vi "DMSP_main_VI_BM.vi"(0 "Constants":T4={"step to ml"=1920.0, "BoardNum"=1, "PosA BitNum"=6, "PosB BitNum"=5, "Heat Pulse Delay (ms)"=0.0, "Heating Iterations"=8, "N rinses"=2, "Dissolution Time (s)"=120, "SpargeBit"=0, "Extra Milli-Q (ml)"=2.0, "Valco Port Number"=6, "BitNum (Thermocouple)"=0, "N syringe rinses"=2, "NaOH Vol (ml)"=2.0, "FanBit"=0}, 1 "Hydrolysis Countdown Refnum":refnum<vi>, 2 "Metadata":T1={"Local save location:"="C:\\Users\\bcamc\\OneDrive\\Desktop\\LabVIEW\\Test_metadata", "Cruise ID"="LaPerouse", "Sampling Timestamp"="2023-07-19 15:23:13", "Elution Timestamp"="2023-07-19 15:29:12", "GPS_Latitude"=-999.0, "GPS_Longitude"=-999.0, "DMS_std_conc"=0.0, "DMSP_std_conc"=0.0, "DMSO_std_conc"=0.0, "Std_index"=0.0, "Initial Trap Temp (oC)"=174.0, "Max Trap Temp (oC)"=174.0, "Final Trap Temp (oC)"=0.0, "Flow Rate (mL/min)"=0.0, "Comment"="", "GPS_Minute"=-999.0, "GPS_Day"=-999.0, "GPS_jd"=-999.0, "GPS_Hour"=-999.0, "GPS_Second"=-999.0, "GPS Baud"=4800.0, "COM Port (GPS)"="COM10", "Use GPS?"=FALSE, "Format Date"="%d-%d-%d"} {"GPS_Latitude" format="%_4g"; "GPS_Longitude" format="%_4g"; "GPS_jd" format="%_5g"; "Std_index" format="%.2g"; "DMSO_std_conc" format="%.2f"; "DMSP_std_conc" format="%.2f"; "DMS_std_conc" format="%.2f"}, 3 "Hydrolysis Progress Bar Refnum":refnum<vi>, 4 "Sparge Countdown Timer Refnum":refnum<vi>, 5 "Sample Params":T5={"DMS Sparge Time (min)"=7.0, "Elution Time (min)"=1.5, "COM port (16 Pos. Valve)"="COM10", "Trap Heating Time (ms)"=675.0, "COM Port (DC Power)"="COM11", "COM Port (Runze)"="COM12", "sample volume"=10.0, "DMSO Red. Duration (min)"=30.0, "Bypass sample handling (debugging)"=FALSE, "Reverse Reduction?"=FALSE, "Voltage (V)"="4.0", "DMSP Hydrolysis Time (min)"=13.0, "Total Vol. (mL)"=12.0, "Split DMSP sample?"=FALSE, "Remove DMSP vol. (mL)"=4.0, "Extra Burn-off"=FALSE}, 6 "Sparging Progress Bar Refnum":refnum<vi>, 7 "Pump Parameters":T3={"Speed 1"="100", "Speed 2"="250", "Speed 3"="450", "Speed 4"="250", "UW/Sample"="5", "Sparge"="2", "Std"="4", "Waste"="15", "Air"="14", "Milli-Q"="1", "H2SO4"="6", "NaOH"="3", "Catalyst"="7", "Cell (H+ side)"="8", "Cell (sample side)"="9", "NaCl"="11"}, 9 "Mode Selection":T2(ring), 10 "Elution Countdown Timer Refnum":refnum<vi>, 11 "Analysis Type":T6(ring)=enum."DMS/P", 12 "Current Analyte Refnum":refnum<vi>, 14 "Temp Refnum":refnum<vi>, 15 "Elution Progress Bar Refnum":refnum<vi>) -> ()   [LabVIEW 2021]
uses:
  SubVIs/Timestamps_global.vi
  SubVIs/Refnum_control_global_BM.vi
  SubVIs/DMSP-related/Hydrolysis_stop.vi
  SubVIs/DMS-related/Sparge_stop.vi
  SubVIs/Plot_trap_heating_global_BM.vi
  SubVIs/DMS-related/Elution_stop.vi
  SubVIs/DMSO-related/Temp_global_BM.vi
panel:
  out "Current Analyte":string
  out "Hydrolysis Countdown (min)":dbl format="%.2g"
  out "Hydrolysis Progress Bar":u8(slide)=100 scale=0.0..100.0
  out "Drying Flow":bool
  out "Heating":bool
  in  "Error in":errorcluster
  out "Sparge Countdown (min)":dbl format="%.2g"
  out "Sparging Progress Bar":u8(slide)=100 scale=0.0..100.0
  out "Temp (oC)":i32=174
  out "Error out":errorcluster
  out "Elution Countdown (min)":dbl format="%.2f"
  out "Sparging":bool
  out "Elution Progress Bar":u8(slide)=100 scale=0.0..100.0
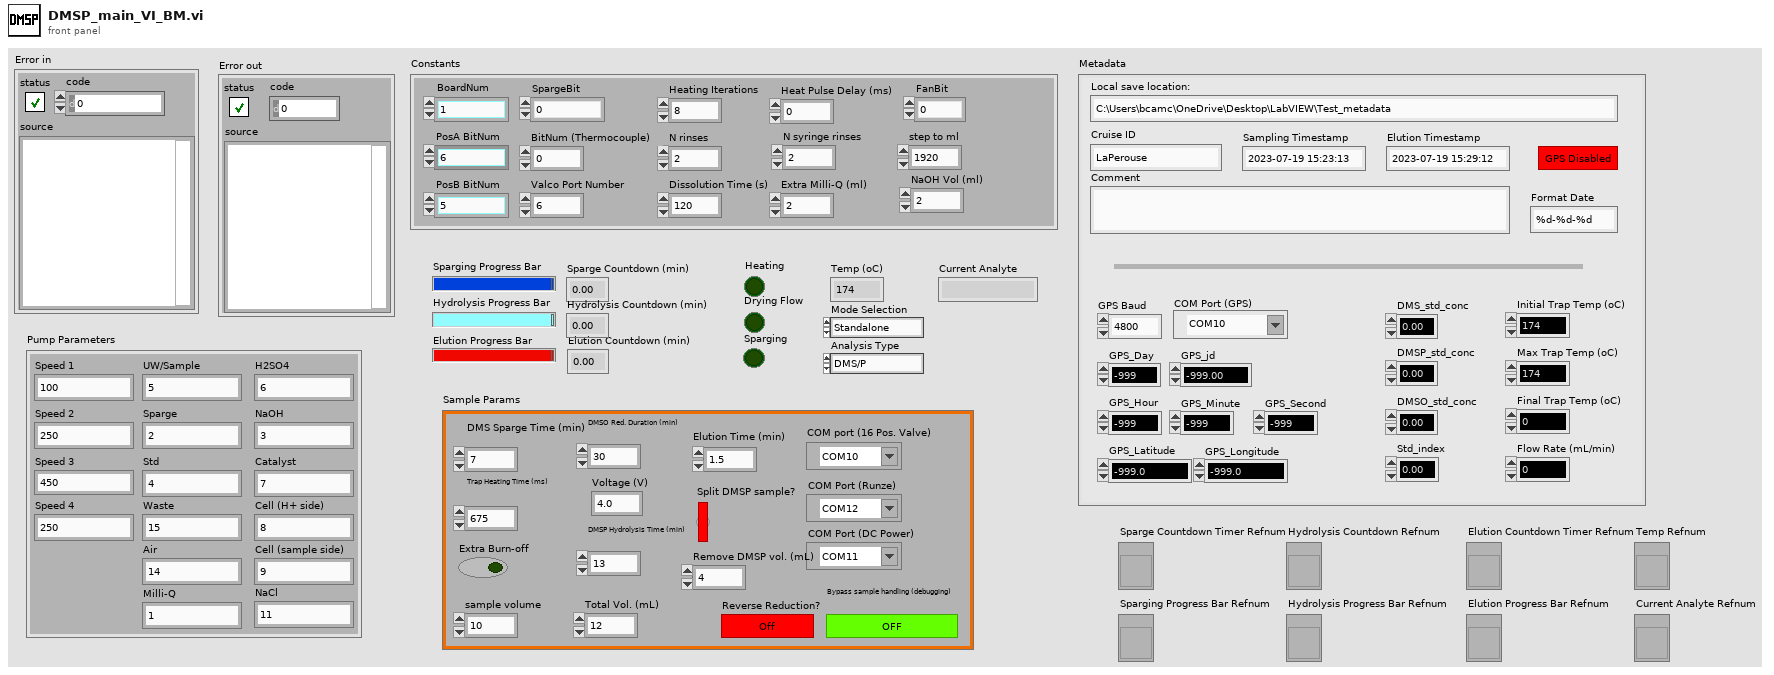
[diagram p1: front panel]
types:
  T1 = cluster{"Local save location:":string, "Cruise ID":string, "Sampling Timestamp":string, "Elution Timestamp":string, "GPS_Latitude":dbl, "GPS_Longitude":dbl, "DMS_std_conc":dbl, "DMSP_std_conc":dbl, "DMSO_std_conc":dbl, "Std_index":dbl, "Initial Trap Temp (oC)":dbl, "Max Trap Temp (oC)":dbl, "Final Trap Temp (oC)":dbl, "Flow Rate (mL/min)":dbl, "Comment":string, "GPS_Minute":dbl, "GPS_Day":dbl, "GPS_jd":dbl, "GPS_Hour":dbl, "GPS_Second":dbl, "GPS Baud":dbl, "COM Port (GPS)":refnum<visa-resource-name>, "Use GPS?":bool, "Format Date":string}
  T2 = enum16{"Standalone", "Analysis", "Standard Curve", "Point Std"}
  T3 = cluster{"Speed 1":string, "Speed 2":string, "Speed 3":string, "Speed 4":string, "UW/Sample":string, "Sparge":string, "Std":string, "Waste":string, "Air":string, "Milli-Q":string, "H2SO4":string, "NaOH":string, "Catalyst":string, "Cell (H+ side)":string, "Cell (sample side)":string, "NaCl":string}
  T4 = cluster{"step to ml":dbl, "BoardNum":u32, "PosA BitNum":u32, "PosB BitNum":u32, "Heat Pulse Delay (ms)":dbl, "Heating Iterations":i32, "N rinses":i32, "Dissolution Time (s)":u32, "SpargeBit":u32, "Extra Milli-Q (ml)":dbl, "Valco Port Number":i32, "BitNum (Thermocouple)":u32, "N syringe rinses":i32, "NaOH Vol (ml)":dbl, "FanBit":u32}
  T5 = cluster{"DMS Sparge Time (min)":dbl, "Elution Time (min)":dbl, "COM port (16 Pos. Valve)":refnum<visa-resource-name>, "Trap Heating Time (ms)":dbl, "COM Port (DC Power)":refnum<visa-resource-name>, "COM Port (Runze)":refnum<visa-resource-name>, "sample volume":dbl, "DMSO Red. Duration (min)":dbl, "Bypass sample handling (debugging)":bool, "Reverse Reduction?":bool, "Voltage (V)":string, "DMSP Hydrolysis Time (min)":dbl, "Total Vol. (mL)":dbl, "Split DMSP sample?":bool, "Remove DMSP vol. (mL)":dbl, "Extra Burn-off":bool}
  T6 = enum16{"DMS Only", "DMS/O", "DMS/P", "DMS/O/P", "DMSO Only"}
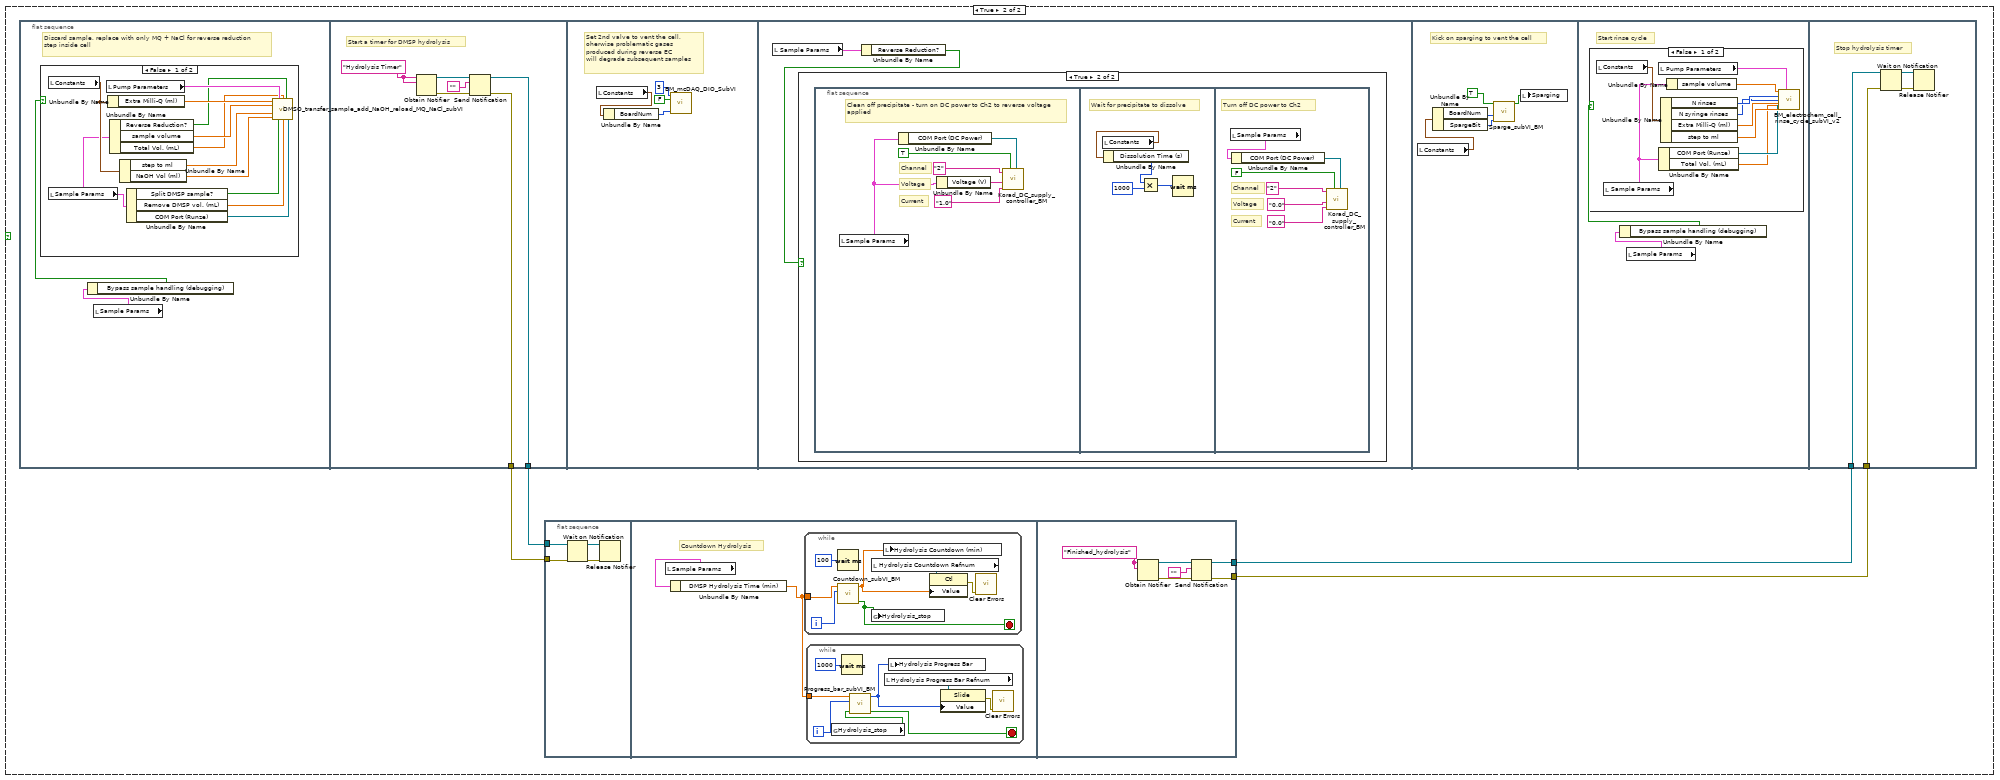
[diagram p10: hidden frame]
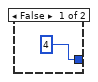
[diagram p15: hidden frame]
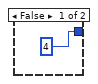
[diagram p17: hidden frame]
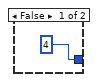
[diagram p20: hidden frame]
diagram:
  n1 = flat-sequence {
    tunnel: [w327] -> w6
    tunnel: [w326] -> w5
    tunnel: [w321] -> w2
    tunnel: [w320] -> w1
    tunnel: [w343] -> w10
    tunnel: [w348] -> w9
    tunnel: w10 -> [w348]
    tunnel: w9 -> [w352]
    tunnel: [w377] -> w8
    tunnel: w8 -> [w387]
    tunnel: [w387] -> w4
    tunnel: w4 -> [w409]
    tunnel: [w409] -> w3
    tunnel: w3 -> [w416]
    tunnel: [w416] -> w7
    tunnel: w7 -> [w424]
    frame #0 {
      w20 = "DMSP" ("Current Analysis")
      # "Update sampling / elution times from DMS VI"
      # "If run on OSSCAR, set the flow path back to the sparge chamber"
      # "Indicate for user to track"
      # "Initalize syringe pump"
      n2 = local read "Constants"() -> (w18:T4)
      n3 = global read "Timestamps_global.vi" "Sampling Timestamp"() -> (w11:string)
      n4 = global read "Timestamps_global.vi" "Elution Timestamp"() -> (w12:string)
      n5 = Unbundle By Name(w18) -> ("BoardNum"=w16:u32)
      n6 = local read "Sample Params"() -> (w22:T5)
      n7 = Unbundle By Name(w22) -> ("Bypass sample handling (debugging)"=w23:bool)
      n8 = case shown="False" w23 {
        frame False {
          n9 = local read "Sample Params"() -> (w26:T5)
          n10 = Unbundle By Name(w26) -> ("COM Port (Runze)"=w27:refnum<visa-resource-name>)
          n11 = call "BM_Runze_Syringe_Pump_Controller.vi"("Initialize Plunger?"=TRUE ("Initialize?"), "COM Port (Runze)"=w27, "Enter Command"="") -> ()  [unwired: 6 in, 3 out]
        }
        frame True {
        }
      }
      n12 = local read "Current Analyte Refnum"() -> (w21:refnum<vi>)
      n13 = local write "Current Analyte"(w20) -> ()
      n14 = Equal?(x=u32 0, y=w16) -> (x = y?=w17:bool)
      n15 = property class="Ctl"(reference=w21, "Value"=w20) -> (error out=w19:errorcluster)  [unwired: 1 in, 1 out]
      n16 = case shown="True" w17 {
        tunnel: w16 -> [_ w24]
        frame False {
        }
        frame True {
          n17 = call "EC_switch_flow_path_subVI_BM.vi"("BoardNum"=w24, "Switch Flow Path"=FALSE) -> ()  [unwired: 10 in]
        }
      }
      n18 = local read "Metadata"() -> (w14:T1)
      n19 = Bundle By Name(cluster=w14, "Sampling Timestamp"=w11, "Elution Timestamp"=w12) -> (w13:T1)
      n20 = call <vilib>:"Clear Errors.vi"("error in (no error)"=w19) -> ()  [unwired: 5 in, 2 out]
      n21 = local write "Metadata"(w13) -> ()
    }
    frame #1 {
      # "Turn on sparging."
      # "Switch Valco valve to position A: load."
      # "Begin sample handling"
      n22 = local read "Constants"() -> (w37:T4)
      n23 = Unbundle By Name(w37) -> ("PosA BitNum"=w36:u32, "PosB BitNum"=w35:u32, "BoardNum"=w34:u32, "SpargeBit"=w33:u32)
      n24 = Equal?(x=w34, y=u32 1) -> (x = y?=w39:bool)
      n25 = case shown="True" w39 {
        tunnel: w34 -> [_ w44]
        frame False {
        }
        frame True {
          # "Switch to sample port"
          # "Start Drying Flow"
          n26 = local read "Constants"() -> (w42:T4)
          n27 = local read "Sample Params"() -> (w40:T5)
          n28 = Unbundle By Name(w40) -> ("COM port (16 Pos. Valve)"=w41:refnum<visa-resource-name>)
          n29 = Unbundle By Name(w42) -> ("Valco Port Number"=w43:i32)
          n30 = call "BM_mcDAQ_DIO_SubVI.vi"("BoardNum"=w44, "BitValue"=TRUE, "BitNum"=4) -> ("Control out"=w47:bool)  [unwired: 8 in]
          n31 = local write "Drying Flow"(w47) -> ()
          n32 = call "16portvalco_subVI_BM.vi"("COM Port (16 Pos. Valve)"=w41, "Port Number"=w43) -> ()  [unwired: 9 in, 1 out]
        }
      }
      n33 = call "Sparge_subVI_BM.vi"("BitNum"=w33, "BoardNum"=w34, "Sparge now"=TRUE) -> ("Sparging"=w38:bool)  [unwired: 8 in]
      n34 = local write "Sparging"(w38) -> ()
      n35 = call "Switch_Valco_6port_subVI_BM.vi"("Load (T) or Inject (F)"=TRUE, "PosA BitNum"=w36, "PosB BitNum"=w35, "BoardNum"=w34) -> ()  [unwired: 6 in, 1 out]
    }
    frame #2 {
      # "2 options here for sampling handling, based on the analysis type:\n1. \"DMS/O/P\" mode - transfer sample to sparger, add NaOH to sparger, start a timer, then either clean off precipitate + rinse cell or just rinse cell, while waiting for hydrolysis to finish\n2. \"DMS/P\" mode - Run DMS VI, split sample (optional), then add NaOH\nOther modes are N/A"
      n36 = local read "Analysis Type"() -> (w50:T6)
      n37 = Equal?(x=w50, y=T6."DMS/O/P") -> (x = y?=w49:bool)
      n38 = case shown="False" w49 {
        frame False {
          n39 = local read "Analysis Type"() -> (w52:T6)
          n40 = Equal?(x=w52, y=T6."DMS/P") -> (x = y?=w51:bool)
          n41 = case shown="True" w51 {
            frame False {
              # "Analysis mode is set to either \"DMS Only\", \"DMSO Only\" or \"DMS/O\", all of which are N/A here"
            }
            frame True {
              n42 = flat-sequence {
                tunnel: [w180] -> w55
                tunnel: [w179] -> w54
                tunnel: w57 -> [w194]
                tunnel: w56 -> [w193]
                frame #0 {
                  # "Sample handle / sparge off DMS first"
                  n43 = while {
                    stop <- w105 stop-if-true
                    # "Update refnums from DMS subVI - this ensures they pass through to main OSSCAR VI"
                    n44 = local read "Elution Countdown Timer Refnum"() -> (w100:refnum<vi>)
                    n45 = local read "Sparge Countdown Timer Refnum"() -> (w112:refnum<vi>)
                    n46 = local read "Elution Countdown Timer Refnum"() -> (w103:refnum<vi>)
                    n47 = local read "Sparging Progress Bar Refnum"() -> (w115:refnum<vi>)
                    n48 = local read "Elution Countdown (min)"() -> (w101:dbl)
                    n49 = local read "Sparge Countdown (min)"() -> (w113:dbl)
                    n50 = local read "Sparging Progress Bar"() -> (w114:u8)
                    n51 = local read "Elution Progress Bar"() -> (w102:u8)
                    n52 = local read "Temp Refnum"() -> (w109:refnum<vi>)
                    n53 = global read "Refnum_control_global_BM.vi" "Refnum_control"() -> (w107:bool)
                    n54 = local read "Temp (oC)"() -> (w108:i32)
                    n55 = property class="Slide"(reference=w115, "Value"=w114) -> (error out=w116:errorcluster)  [unwired: 1 in, 1 out]
                    n56 = property class="Ctl"(reference=w100, "Value"=w101) -> (error out=w99:errorcluster)  [unwired: 1 in, 1 out]
                    n57 = property class="Ctl"(reference=w109, "Value"=w108) -> (error out=w110:errorcluster)  [unwired: 1 in, 1 out]
                    n58 = property class="Ctl"(reference=w112, "Value"=w113) -> (error out=w111:errorcluster)  [unwired: 1 in, 1 out]
                    n59 = property class="Ctl"(reference=w103, "Value"=w102) -> (error out=w104:errorcluster)  [unwired: 1 in, 1 out]
                    n60 = Equal?(x=w107, y=TRUE) -> (x = y?=w105:bool)
                    n61 = call <vilib>:"Clear Errors.vi"("error in (no error)"=w116) -> ()  [unwired: 5 in, 2 out]
                    n62 = call <vilib>:"Clear Errors.vi"("error in (no error)"=w99) -> ()  [unwired: 5 in, 2 out]
                    n63 = call <vilib>:"Clear Errors.vi"("error in (no error)"=w110) -> ()  [unwired: 5 in, 2 out]
                    n64 = Wait (ms)(milliseconds to wait=u32 100) -> ()  [unwired: 1 out]
                    n65 = call <vilib>:"Clear Errors.vi"("error in (no error)"=w111) -> ()  [unwired: 5 in, 2 out]
                    n66 = call <vilib>:"Clear Errors.vi"("error in (no error)"=w104) -> ()  [unwired: 5 in, 2 out]
                  }
                  n67 = local read "Pump Parameters"() -> (w95:T3)
                  n68 = local read "Mode Selection"() -> (w87:T2)
                  n69 = local read "Sample Params"() -> (w96:T5)
                  n70 = local read "Analysis Type"() -> (w94:T6)
                  n71 = local read "Constants"() -> (w97:T4)
                  n72 = local read "Metadata"() -> (w93:T1)
                  n73 = control-ref of="Elution Countdown (min)"() -> (w90:refnum<vi>)
                  n74 = control-ref of="Temp (oC)"() -> (w89:refnum<vi>)
                  n75 = control-ref of="Current Analyte"() -> (w85:refnum<vi>)
                  n76 = control-ref of="Elution Progress Bar"() -> (w91:refnum<vi>)
                  n77 = control-ref of="Sparge Countdown (min)"() -> (w92:refnum<vi>)
                  n78 = control-ref of="Sparging Progress Bar"() -> (w88:refnum<vi>)
                  n79 = call "DMS_main_VI_BM.vi"("Constants"=w97, "Metadata"=w93, "Skip sample handling"=FALSE, "Sparging Countdown Timer Refnum"=w92, "Sample Params"=w96, "Sparging Progress Bar Refnum"=w88, "Pump Parameters"=w95, "Mode Selection"=w87, "Elution Countdown Timer Refnum"=w90, "Analysis Type"=w94, "Current Analyte Refnum"=w85, "Temp Refnum"=w89, "Elution Progress Bar Refnum"=w91) -> ()  [unwired: 3 in]
                }
                frame #1 {
                  # "Optional: If splitting DMSP sample to reduce ion counts on the detector, remove chosen vol. here and send to waste"
                  n80 = local read "Sample Params"() -> (w118:T5)
                  n81 = Unbundle By Name(w118) -> ("Split DMSP sample?"=w117:bool)
                  n82 = case shown="True" w117 {
                    frame False {
                      # "If not splitting sample, continue with analysis"
                    }
                    frame True {
                      n83 = local read "Sample Params"() -> (w124:T5)
                      n84 = local read "Pump Parameters"() -> (w136:T3)
                      n85 = local read "Constants"() -> (w122:T4)
                      n86 = Unbundle By Name(w124) -> ("Remove DMSP vol. (mL)"=w125:dbl)
                      n87 = Unbundle By Name(w124) -> ("Remove DMSP vol. (mL)"=w126:dbl)
                      n88 = Unbundle By Name(w122) -> ("step to ml"=w121:dbl)
                      n89 = Unbundle By Name(w122) -> ("step to ml"=w123:dbl)
                      n90 = Multiply(x=w125, y=w121) -> (x*y=w146:dbl)
                      n91 = Multiply(x=w126, y=w123) -> (x*y=w148:dbl)
                      n92 = Unbundle By Name(w136) -> ("Speed 2"=w139:string)
                      n93 = Unbundle By Name(w136) -> ("Speed 1"=w149:string)
                      n94 = Unbundle By Name(w136) -> ("Sparge"=w135:string)
                      n95 = Unbundle By Name(w136) -> ("Waste"=w134:string)
                      n96 = Number To Decimal String(number=w148) -> (decimal integer string=w147:string)  [unwired: 1 out]
                      n97 = Number To Decimal String(number=w146) -> (decimal integer string=w145:string)  [unwired: 1 out]
                      n98 = Concatenate Strings("V", w149) -> (w144:string)
                      n99 = Concatenate Strings("O", w135) -> (w143:string)
                      n100 = Concatenate Strings("P", w147) -> (w142:string)
                      n101 = Concatenate Strings("O", w134) -> (w141:string)
                      n102 = Concatenate Strings("D", w145) -> (w137:string)
                      n103 = Concatenate Strings("V", w139) -> (w138:string)
                      n104 = local read "Sample Params"() -> (w119:T5)
                      n105 = Unbundle By Name(w119) -> ("COM Port (Runze)"=w120:refnum<visa-resource-name>)
                      n106 = Concatenate Strings(w144, w143, w142, w141, w138, w137) -> (w140:string)
                      n107 = call "BM_Runze_Syringe_Pump_Controller.vi"("Initialize Plunger?"=FALSE ("Initialize?"), "COM Port (Runze)"=w120, "Enter Command"=w140) -> ()  [unwired: 6 in, 3 out]
                    }
                  }
                }
                frame #2 {
                  # "Turn on sparging."
                  # "Switch Valco valve to position A: load."
                  # "Begin sample handling"
                  n108 = local read "Constants"() -> (w158:T4)
                  n109 = Unbundle By Name(w158) -> ("PosA BitNum"=w157:u32, "PosB BitNum"=w156:u32, "BoardNum"=w155:u32, "SpargeBit"=w154:u32)
                  n110 = Equal?(x=w155, y=u32 1) -> (x = y?=w150:bool)
                  n111 = case shown="True" w150 {
                    tunnel: w155 -> [_ w164]
                    frame False {
                    }
                    frame True {
                      # "Switch to sample port"
                      # "Start Drying Flow"
                      n112 = local read "Constants"() -> (w162:T4)
                      n113 = local read "Sample Params"() -> (w160:T5)
                      n114 = Unbundle By Name(w160) -> ("COM port (16 Pos. Valve)"=w161:refnum<visa-resource-name>)
                      n115 = Unbundle By Name(w162) -> ("Valco Port Number"=w163:i32)
                      n116 = call "BM_mcDAQ_DIO_SubVI.vi"("BoardNum"=w164, "BitValue"=TRUE, "BitNum"=4) -> ("Control out"=w167:bool)  [unwired: 8 in]
                      n117 = local write "Drying Flow"(w167) -> ()
                      n118 = call "16portvalco_subVI_BM.vi"("COM Port (16 Pos. Valve)"=w161, "Port Number"=w163) -> ()  [unwired: 9 in, 1 out]
                    }
                  }
                  n119 = call "Sparge_subVI_BM.vi"("BitNum"=w154, "BoardNum"=w155, "Sparge now"=TRUE) -> ("Sparging"=w159:bool)  [unwired: 8 in]
                  n120 = local write "Sparging"(w159) -> ()
                  n121 = call "Switch_Valco_6port_subVI_BM.vi"("Load (T) or Inject (F)"=TRUE, "PosA BitNum"=w157, "PosB BitNum"=w156, "BoardNum"=w155) -> ()  [unwired: 6 in, 1 out]
                }
                frame #3 {
                  # "Add NaOH to sparger"
                  n122 = local read "Sample Params"() -> (w168:T5)
                  n123 = Unbundle By Name(w168) -> ("Bypass sample handling (debugging)"=w169:bool)
                  n124 = case shown="False" w169 {
                    frame False {
                      n125 = local read "Sample Params"() -> (w173:T5)
                      n126 = local read "Sample Params"() -> (w175:T5)
                      n127 = local read "Constants"() -> (w177:T4)
                      n128 = local read "Pump Parameters"() -> (w178:T3)
                      n129 = Unbundle By Name(w177) -> ("step to ml"=w176:dbl, "NaOH Vol (ml)"=w171:dbl)
                      n130 = Unbundle By Name(w173) -> ("COM Port (Runze)"=w172:refnum<visa-resource-name>)
                      n131 = Unbundle By Name(w175) -> ("sample volume"=w174:dbl, "Total Vol. (mL)"=w170:dbl)
                      n132 = call "DMSP_add_NaOH_BM.vi"("COM Port"=w172, "Pump Parameters"=w178, "NaOH Vol (mL)"=w171, "step to ml"=w176, "Total Vol. (mL)"=w170, "Sample Vol. (mL)"=w174) -> ()  [unwired: 6 in]
                    }
                    frame True {
                    }
                  }
                }
                frame #4 {
                  w181 = "Hydrolysis Timer"
                  # "Start a timer for DMSP hydrolysis"
                  n133 = Obtain Notifier(name (unnamed)=w181, notification data type=w181) -> (notifier out=w183:refnum<notifier>, error out=w184:errorcluster)  [unwired: 2 in, 1 out]
                  n134 = Send Notification(notification="", notifier=w183, error in (no error)=w184) -> (notifier out=w180:refnum<notifier>, error out=w179:errorcluster)
                }
                frame #5 {
                  # "Rinse Syringe"
                  n135 = local read "Sample Params"() -> (w185:T5)
                  n136 = Unbundle By Name(w185) -> ("Bypass sample handling (debugging)"=w186:bool)
                  n137 = case shown="False" w186 {
                    frame False {
                      n138 = local read "Sample Params"() -> (w189:T5)
                      n139 = local read "Constants"() -> (w191:T4)
                      n140 = local read "Pump Parameters"() -> (w192:T3)
                      n141 = Unbundle By Name(w191) -> ("step to ml"=w190:dbl, "N syringe rinses"=w187:i32)
                      n142 = Unbundle By Name(w189) -> ("COM Port (Runze)"=w188:refnum<visa-resource-name>)
                      n143 = call "Rinse_syringe_subVI_BM.vi"("COM Port"=w188, "Pump Parameters"=w192, "N syringe rinses"=w187, "step to ml"=w190) -> ()  [unwired: 8 in]
                    }
                    frame True {
                    }
                  }
                }
                frame #6 {
                  # "Stop hydrolysis timer"
                  n144 = Wait on Notification(notifier=w194, error in (no error)=w193) -> (notifier out=w195:refnum<notifier>, error out=w196:errorcluster)  [unwired: 4 out]
                  n145 = Release Notifier(notifier=w195, error in (no error)=w196) -> ()  [unwired: 1 in, 3 out]
                }
              }
              n146 = flat-sequence {
                tunnel: w54 -> [w58]
                tunnel: w55 -> [w59]
                tunnel: [w80] -> w57
                tunnel: [w79] -> w56
                frame #0 {
                  n147 = Wait on Notification(notifier=w59, error in (no error)=w58) -> (notifier out=w61:refnum<notifier>, error out=w60:errorcluster)  [unwired: 4 out]
                  n148 = Release Notifier(notifier=w61, error in (no error)=w60) -> ()  [unwired: 1 in, 3 out]
                }
                frame #1 {
                  # "Countdown Hydrolysis"
                  n149 = local read "Sample Params"() -> (w63:T5)
                  n150 = Unbundle By Name(w63) -> ("DMSP Hydrolysis Time (min)"=w62:dbl)
                  n151 = while {
                    tunnel: w62 -> [w77]
                    i -> [w76]
                    stop <- w75 stop-if-true
                    n152 = Wait (ms)(milliseconds to wait=u32 100) -> ()  [unwired: 1 out]
                    n153 = call "Countdown_subVI_BM.vi"("Current Iteration"=w76, "Runtime (min)"=w77) -> ("Global Stop"=w75:bool, "Countdown Timer (min)"=w74:dbl)  [unwired: 8 in]
                    n154 = global write "Hydrolysis_stop.vi" "Hydrolysis_stop"(w75) -> ()
                    n155 = local read "Hydrolysis Countdown Refnum"() -> (w72:refnum<vi>)
                    n156 = local write "Hydrolysis Countdown (min)"(w74) -> ()
                    n157 = property class="Ctl"(reference=w72, "Value"=w74) -> (error out=w73:errorcluster)  [unwired: 1 in, 1 out]
                    n158 = call <vilib>:"Clear Errors.vi"("error in (no error)"=w73) -> ()  [unwired: 5 in, 2 out]
                  }
                  n159 = while {
                    tunnel: w62 -> [w70]
                    i -> [w69]
                    stop <- w67 stop-if-true
                    n160 = global read "Hydrolysis_stop.vi" "Hydrolysis_stop"() -> (w68:bool)
                    n161 = Wait (ms)(milliseconds to wait=u32 1000) -> ()  [unwired: 1 out]
                    n162 = call "Progress_bar_subVI_BM.vi"("Global Stop"=w68, "Current Iteration"=w69, "Runtime (min)"=w70) -> ("Loop Stop"=w67:bool, "Progress Bar"=w66:u8)  [unwired: 7 in]
                    n163 = local read "Hydrolysis Progress Bar Refnum"() -> (w64:refnum<vi>)
                    n164 = local write "Hydrolysis Progress Bar"(w66) -> ()
                    n165 = property class="Slide"(reference=w64, "Value"=w66) -> (error out=w65:errorcluster)  [unwired: 1 in, 1 out]
                    n166 = call <vilib>:"Clear Errors.vi"("error in (no error)"=w65) -> ()  [unwired: 5 in, 2 out]
                  }
                }
                frame #2 {
                  w83 = "Finished_hydrolysis"
                  n167 = Obtain Notifier(name (unnamed)=w83, notification data type=w83) -> (notifier out=w81:refnum<notifier>, error out=w82:errorcluster)  [unwired: 2 in, 1 out]
                  n168 = Send Notification(notification="", notifier=w81, error in (no error)=w82) -> (notifier out=w80:refnum<notifier>, error out=w79:errorcluster)
                }
              }
            }
          }
        }
        frame True {
          n169 = flat-sequence {
            tunnel: [w244] -> w200
            tunnel: [w243] -> w199
            tunnel: w197 -> [w288]
            tunnel: w198 -> [w287]
            frame #0 {
              # "Discard sample, replace with only MQ + NaCl for reverse reduction step inside cell"
              n170 = local read "Sample Params"() -> (w229:T5)
              n171 = Unbundle By Name(w229) -> ("Bypass sample handling (debugging)"=w228:bool)
              n172 = case shown="False" w228 {
                frame False {
                  n173 = local read "Constants"() -> (w239:T4)
                  n174 = local read "Sample Params"() -> (w237:T5)
                  n175 = local read "Pump Parameters"() -> (w241:T3)
                  n176 = Unbundle By Name(w239) -> ("Extra Milli-Q (ml)"=w240:dbl)
                  n177 = Unbundle By Name(w237) -> ("Reverse Reduction?"=w233:bool, "sample volume"=w238:dbl, "Total Vol. (mL)"=w232:dbl)
                  n178 = Unbundle By Name(w239) -> ("step to ml"=w235:dbl, "NaOH Vol (ml)"=w234:dbl)
                  n179 = Unbundle By Name(w237) -> ("Split DMSP sample?"=w230:bool, "Remove DMSP vol. (mL)"=w231:dbl, "COM Port (Runze)"=w236:refnum<visa-resource-name>)
                  n180 = call "DMSO_transfer_sample_add_NaOH_reload_MQ_NaCl_subVI.vi"("Extra Milli-Q (ml)"=w240, "Pump Parameters"=w241, "Total Vol. (mL)"=w232, "Reverse Reduction?"=w233, "Sample Vol. (mL)"=w238, "step to ml"=w235, "NaOH Vol (mL)"=w234, "Split DMSP sample?"=w230, "Remove DMSP vol. (mL)"=w231, "COM Port"=w236) -> ()  [unwired: 6 in]
                }
                frame True {
                }
              }
            }
            frame #1 {
              w245 = "Hydrolysis Timer"
              # "Start a timer for DMSP hydrolysis"
              n181 = Obtain Notifier(name (unnamed)=w245, notification data type=w245) -> (notifier out=w246:refnum<notifier>, error out=w247:errorcluster)  [unwired: 2 in, 1 out]
              n182 = Send Notification(notification="", notifier=w246, error in (no error)=w247) -> (notifier out=w243:refnum<notifier>, error out=w244:errorcluster)
            }
            frame #2 {
              # "Set 2nd valve to vent the cell,\noherwise problematic gases\nproduced during reverse EC \nwill degrade subsequent samples"
              n183 = local read "Constants"() -> (w248:T4)
              n184 = Unbundle By Name(w248) -> ("BoardNum"=w251:u32)
              n185 = call "BM_mcDAQ_DIO_SubVI.vi"("BoardNum"=w251, "BitValue"=FALSE, "BitNum"=u32 3) -> ()  [unwired: 8 in, 1 out]
            }
            frame #3 {
              n186 = local read "Sample Params"() -> (w253:T5)
              n187 = Unbundle By Name(w253) -> ("Reverse Reduction?"=w252:bool)
              n188 = case shown="True" w252 {
                frame False {
                  # "Skip to rinsing out the cell"
                }
                frame True {
                  n189 = flat-sequence {
                    frame #0 {
                      # "Channel"
                      # "Current"
                      # "Voltage"
                      # "Clean off precipitate - turn on DC power to Ch2 to reverse voltage applied"
                      n190 = local read "Sample Params"() -> (w254:T5)
                      n191 = Unbundle By Name(w254) -> ("COM Port (DC Power)"=w256:refnum<visa-resource-name>)
                      n192 = Unbundle By Name(w254) -> ("Voltage (V)"=w255:string)
                      n193 = call "Korad_DC_supply_controller_BM.vi"("COM Port"=w256, "Master Output Control"=TRUE ("Output Control"), "Current"="1.0" ("Ch2 Current"), "Voltage"=w255, "Channel"="2" ("Ch1 Voltage")) -> ()  [unwired: 7 in]
                    }
                    frame #1 {
                      # "Wait for precipitate to dissolve"
                      n194 = local read "Constants"() -> (w261:T4)
                      n195 = Unbundle By Name(w261) -> ("Dissolution Time (s)"=w260:u32)
                      n196 = Multiply(x=w260, y=u32 1000) -> (x*y=w263:u32)
                      n197 = Wait (ms)(milliseconds to wait=w263) -> ()  [unwired: 1 out]
                    }
                    frame #2 {
                      # "Channel"
                      # "Current"
                      # "Voltage"
                      # "Turn off DC power to Ch2"
                      n198 = local read "Sample Params"() -> (w265:T5)
                      n199 = Unbundle By Name(w265) -> ("COM Port (DC Power)"=w264:refnum<visa-resource-name>)
                      n200 = call "Korad_DC_supply_controller_BM.vi"("COM Port"=w264, "Master Output Control"=FALSE ("Output Control"), "Current"="0.0" ("Ch2 Current"), "Voltage"="0.0" ("Ch1 Voltage"), "Channel"="2" ("Ch1 Voltage")) -> ()  [unwired: 7 in]
                    }
                  }
                }
              }
            }
            frame #4 {
              # "Kick on sparging to vent the cell"
              n201 = local read "Constants"() -> (w272:T4)
              n202 = Unbundle By Name(w272) -> ("BoardNum"=w271:u32, "SpargeBit"=w270:u32)
              n203 = call "Sparge_subVI_BM.vi"("BitNum"=w270, "BoardNum"=w271, "Sparge now"=TRUE) -> ("Sparging"=w273:bool)  [unwired: 8 in]
              n204 = local write "Sparging"(w273) -> ()
            }
            frame #5 {
              # "Start rinse cycle"
              n205 = local read "Sample Params"() -> (w275:T5)
              n206 = Unbundle By Name(w275) -> ("Bypass sample handling (debugging)"=w276:bool)
              n207 = case shown="False" w276 {
                frame False {
                  n208 = local read "Constants"() -> (w283:T4)
                  n209 = local read "Sample Params"() -> (w280:T5)
                  n210 = local read "Pump Parameters"() -> (w286:T3)
                  n211 = Unbundle By Name(w280) -> ("COM Port (Runze)"=w281:refnum<visa-resource-name>, "Total Vol. (mL)"=w277:dbl)
                  n212 = Unbundle By Name(w283) -> ("N rinses"=w279:i32, "N syringe rinses"=w278:i32, "Extra Milli-Q (ml)"=w285:dbl, "step to ml"=w284:dbl)
                  n213 = Unbundle By Name(w280) -> ("sample volume"=w282:dbl)
                  n214 = call "BM_electrochem_cell_rinse_cycle_subVI_v2.vi"("Sample Volume"=w282, "Pump Parameters"=w286, "N cell rinses"=w279, "N syringe rinses"=w278, "Extra Milli-Q (ml)"=w285, "step to ml"=w284, "COM Port"=w281, "Total Vol. (mL)"=w277) -> ()  [unwired: 8 in]
                }
                frame True {
                }
              }
            }
            frame #6 {
              # "Stop hydrolysis timer"
              n215 = Wait on Notification(notifier=w287, error in (no error)=w288) -> (notifier out=w289:refnum<notifier>, error out=w290:errorcluster)  [unwired: 4 out]
              n216 = Release Notifier(notifier=w289, error in (no error)=w290) -> ()  [unwired: 1 in, 3 out]
            }
          }
          n217 = flat-sequence {
            tunnel: w200 -> [w201]
            tunnel: w199 -> [w202]
            tunnel: [w223] -> w198
            tunnel: [w222] -> w197
            frame #0 {
              n218 = Wait on Notification(notifier=w202, error in (no error)=w201) -> (notifier out=w204:refnum<notifier>, error out=w203:errorcluster)  [unwired: 4 out]
              n219 = Release Notifier(notifier=w204, error in (no error)=w203) -> ()  [unwired: 1 in, 3 out]
            }
            frame #1 {
              # "Countdown Hydrolysis"
              n220 = local read "Sample Params"() -> (w206:T5)
              n221 = Unbundle By Name(w206) -> ("DMSP Hydrolysis Time (min)"=w205:dbl)
              n222 = while {
                tunnel: w205 -> [w220]
                i -> [w219]
                stop <- w218 stop-if-true
                n223 = Wait (ms)(milliseconds to wait=u32 100) -> ()  [unwired: 1 out]
                n224 = call "Countdown_subVI_BM.vi"("Current Iteration"=w219, "Runtime (min)"=w220) -> ("Global Stop"=w218:bool, "Countdown Timer (min)"=w217:dbl)  [unwired: 8 in]
                n225 = global write "Hydrolysis_stop.vi" "Hydrolysis_stop"(w218) -> ()
                n226 = local read "Hydrolysis Countdown Refnum"() -> (w215:refnum<vi>)
                n227 = local write "Hydrolysis Countdown (min)"(w217) -> ()
                n228 = property class="Ctl"(reference=w215, "Value"=w217) -> (error out=w216:errorcluster)  [unwired: 1 in, 1 out]
                n229 = call <vilib>:"Clear Errors.vi"("error in (no error)"=w216) -> ()  [unwired: 5 in, 2 out]
              }
              n230 = while {
                tunnel: w205 -> [w213]
                i -> [w212]
                stop <- w210 stop-if-true
                n231 = global read "Hydrolysis_stop.vi" "Hydrolysis_stop"() -> (w211:bool)
                n232 = Wait (ms)(milliseconds to wait=u32 1000) -> ()  [unwired: 1 out]
                n233 = call "Progress_bar_subVI_BM.vi"("Global Stop"=w211, "Current Iteration"=w212, "Runtime (min)"=w213) -> ("Loop Stop"=w210:bool, "Progress Bar"=w209:u8)  [unwired: 7 in]
                n234 = local read "Hydrolysis Progress Bar Refnum"() -> (w207:refnum<vi>)
                n235 = local write "Hydrolysis Progress Bar"(w209) -> ()
                n236 = property class="Slide"(reference=w207, "Value"=w209) -> (error out=w208:errorcluster)  [unwired: 1 in, 1 out]
                n237 = call <vilib>:"Clear Errors.vi"("error in (no error)"=w208) -> ()  [unwired: 5 in, 2 out]
              }
            }
            frame #2 {
              w226 = "Finished_hydrolysis"
              n238 = Obtain Notifier(name (unnamed)=w226, notification data type=w226) -> (notifier out=w224:refnum<notifier>, error out=w225:errorcluster)  [unwired: 2 in, 1 out]
              n239 = Send Notification(notification="", notifier=w224, error in (no error)=w225) -> (notifier out=w223:refnum<notifier>, error out=w222:errorcluster)
            }
          }
        }
      }
    }
    frame #3 {
      # "Countdown sparging"
      n240 = local read "Sample Params"() -> (w291:T5)
      n241 = Unbundle By Name(w291) -> ("DMS Sparge Time (min)"=w292:dbl)
      n242 = while {
        tunnel: w292 -> [w306]
        i -> [w305]
        stop <- w304 stop-if-true
        n243 = Wait (ms)(milliseconds to wait=u32 100) -> ()  [unwired: 1 out]
        n244 = call "Countdown_subVI_BM.vi"("Current Iteration"=w305, "Runtime (min)"=w306) -> ("Global Stop"=w304:bool, "Countdown Timer (min)"=w302:dbl)  [unwired: 8 in]
        n245 = global write "Sparge_stop.vi" "Sparge_stop"(w304) -> ()
        n246 = local write "Sparge Countdown (min)"(w302) -> ()
        n247 = property class="Ctl"(reference="Sparge Countdown Timer Refnum", "Value"=w302) -> (error out=w301:errorcluster)  [unwired: 1 in, 1 out]
        n248 = call <vilib>:"Clear Errors.vi"("error in (no error)"=w301) -> ()  [unwired: 5 in, 2 out]
      }
      n249 = while {
        tunnel: w292 -> [w299]
        i -> [w298]
        stop <- w296 stop-if-true
        n250 = global read "Sparge_stop.vi" "Sparge_stop"() -> (w297:bool)
        n251 = Wait (ms)(milliseconds to wait=u32 1000) -> ()  [unwired: 1 out]
        n252 = call "Progress_bar_subVI_BM.vi"("Global Stop"=w297, "Current Iteration"=w298, "Runtime (min)"=w299) -> ("Loop Stop"=w296:bool, "Progress Bar"=w294:u8)  [unwired: 7 in]
        n253 = local write "Sparging Progress Bar"(w294) -> ()
        n254 = property class="Slide"(reference="Sparging Progress Bar Refnum", "Value"=w294) -> (error out=w293:errorcluster)  [unwired: 1 in, 1 out]
        n255 = call <vilib>:"Clear Errors.vi"("error in (no error)"=w293) -> ()  [unwired: 5 in, 2 out]
      }
    }
    frame #4 {
      # "Turn off sparging"
      n256 = local read "Constants"() -> (w310:T4)
      n257 = Unbundle By Name(w310) -> ("BoardNum"=w308:u32, "SpargeBit"=w309:u32)
      n258 = Equal?(x=w308, y=u32 1) -> (x = y?=w313:bool)
      n259 = case shown="True" w313 {
        tunnel: w308 -> [_ w316]
        frame False {
        }
        frame True {
          # "Stop Drying Flow"
          n260 = call "BM_mcDAQ_DIO_SubVI.vi"("BoardNum"=w316, "BitValue"=FALSE, "BitNum"=4) -> ("Control out"=w317:bool)  [unwired: 8 in]
          n261 = local write "Drying Flow"(w317) -> ()
        }
      }
      n262 = global write "Sparge_stop.vi" "Sparge_stop"(FALSE ("Stop_Reached")) -> ()
      n263 = call "Sparge_subVI_BM.vi"("BitNum"=w309, "BoardNum"=w308, "Sparge now"=FALSE) -> ("Sparging"=w312:bool)  [unwired: 8 in]
      n264 = local write "Sparging"(w312) -> ()
    }
    frame #5 {
      w322 = "Start_rinsing"
      w329 = "Plot_trap_heating"
      # "Trigger plot in main VI"
      # "Trigger plot in main VI"
      # "Pause to let sparge\npressure dissipate\n\n(Set to 0 for now since this is done in the sparging subVI already)"
      n265 = Obtain Notifier(name (unnamed)=w322, notification data type=w322) -> (notifier out=w325:refnum<notifier>, error out=w324:errorcluster)  [unwired: 2 in, 1 out]
      n266 = global write "Plot_trap_heating_global_BM.vi" "Plot trap heating"(TRUE ("Plot trap heating")) -> ()
      n267 = Wait (ms)(milliseconds to wait=10000) -> ()  [unwired: 1 out]
      n268 = Obtain Notifier(name (unnamed)=w329, notification data type=w329) -> (notifier out=w331:refnum<notifier>, error out=w332:errorcluster)  [unwired: 2 in, 1 out]
      n269 = global write "Plot_trap_heating_global_BM.vi" "Plot trap heating"(TRUE ("Plot trap heating")) -> ()
      n270 = Send Notification(notification="", notifier=w325, error in (no error)=w324) -> (notifier out=w321:refnum<notifier>, error out=w320:errorcluster)
      n271 = Send Notification(notification="", notifier=w331, error in (no error)=w332) -> (notifier out=w327:refnum<notifier>, error out=w326:errorcluster)
    }
    frame #6 {
      # "Turn front panel indicator on"
      # "Apply heat test - does trap heat correctly?"
      n272 = local read "Constants"() -> (w339:T4)
      n273 = local read "Sample Params"() -> (w337:T5)
      n274 = Unbundle By Name(w337) -> ("Trap Heating Time (ms)"=w336:dbl)
      n275 = local read "Error in"() -> (w342:errorcluster)
      n276 = Unbundle By Name(w339) -> ("BoardNum"=w338:u32, "BitNum (Thermocouple)"=w335:u32)
      n277 = local write "Heating"(TRUE ("Heating")) -> ()
      n278 = call "BM_heat_test_subVI.vi"("error in (no error)"=w342, "Heat Pulse Delay (ms)"=u32 1000, "Trap Heating Time (ms)"=w336, "BitNum"=w335, "BoardNum"=w338) -> ("error out"=w343:errorcluster)  [unwired: 6 out]
    }
    frame #7 {
      # "Set valve to inject (pos B)"
      n279 = local read "Constants"() -> (w347:T4)
      n280 = Unbundle By Name(w347) -> ("PosA BitNum"=w346:u32, "PosB BitNum"=w345:u32, "BoardNum"=w344:u32)
      n281 = call "Switch_Valco_6port_subVI_BM.vi"("Load (T) or Inject (F)"=FALSE, "PosA BitNum"=w346, "PosB BitNum"=w345, "BoardNum"=w344) -> ()  [unwired: 6 in, 1 out]
    }
    frame #8 {
      # "Loop to heat trap - pulsing timer can be changed to modulate heating"
      n282 = local read "Constants"() -> (w351:T4)
      n283 = Unbundle By Name(w351) -> ("Heating Iterations"=w350:i32)
      n284 = for {
        N: w350 -> [_]
        tunnel: w352 -> [w356]
        n285 = flat-sequence {
          tunnel: [w361] -> w354
          tunnel: [w359] -> w353
          tunnel: w356 -> [w361]
          tunnel: [w365] -> w355
          tunnel: w354 -> [w365]
          tunnel: w353 -> [w364]
          tunnel: w355 -> [w368]
          frame #0 {
            # "Apply current"
            n286 = local read "Constants"() -> (w360:T4)
            n287 = local read "Sample Params"() -> (w357:T5)
            n288 = Unbundle By Name(w357) -> ("Trap Heating Time (ms)"=w358:dbl)
            n289 = Unbundle By Name(w360) -> ("BoardNum"=w359:u32)
            n290 = call "BM_mcDAQ_DIO_SubVI.vi"("BoardNum"=w359, "BitValue"=TRUE, "BitNum"=7) -> ()  [unwired: 8 in, 1 out]
            n291 = Wait (ms)(milliseconds to wait=w358) -> ()  [unwired: 1 out]
          }
          frame #1 {
            # "Stop current"
            n292 = call "BM_mcDAQ_DIO_SubVI.vi"("BoardNum"=w364, "BitValue"=FALSE, "BitNum"=7) -> ()  [unwired: 8 in, 1 out]
          }
          frame #2 {
            # "\"Pulse\" wait timer"
            n293 = local read "Constants"() -> (w370:T4)
            n294 = Unbundle By Name(w370) -> ("Heat Pulse Delay (ms)"=w369:dbl)
            n295 = local write "Error out"(w368) -> ()
            n296 = Wait (ms)(milliseconds to wait=w369) -> ()  [unwired: 1 out]
          }
        }
      }
    }
    frame #9 {
      # "Wait For Trap\nto reach\nMax Temp \nbefore Cooling"
      n297 = Wait (ms)(milliseconds to wait=10000) -> ()  [unwired: 1 out]
    }
    frame #10 {
      # "Turn on fan"
      # "Turn front panel indicator off"
      # "Start drying flow again"
      n298 = local read "Constants"() -> (w373:T4)
      n299 = Unbundle By Name(w373) -> ("BoardNum"=w372:u32)
      n300 = Equal?(x=w372, y=u32 1) -> (x = y?=w377:bool)
      n301 = local write "Heating"(FALSE ("Heating")) -> ()
      n302 = case shown="True" w377 {
        tunnel: w372 -> [_ w382]
        frame False {
        }
        frame True {
          n303 = call "BM_mcDAQ_DIO_SubVI.vi"("BoardNum"=w382, "BitValue"=TRUE, "BitNum"=u32 4) -> ("Control out"=w381:bool)  [unwired: 8 in]
          n304 = local write "Drying Flow"(w381) -> ()
        }
      }
      n305 = case shown="True" w377 {
        tunnel: [u32 4 ("BitNum") u32 2 ("BitNum")] -> w375
        frame False {
        }
        frame True {
        }
      }
      n306 = call "BM_mcDAQ_DIO_SubVI.vi"("BoardNum"=w372, "BitValue"=TRUE, "BitNum"=w375) -> ()  [unwired: 8 in, 1 out]
    }
    frame #11 {
      # "Elution - allow time for gas to pass through GC column"
      n307 = local read "Sample Params"() -> (w386:T5)
      n308 = Unbundle By Name(w386) -> ("Elution Time (min)"=w385:dbl)
      n309 = while {
        tunnel: w385 -> [w401]
        i -> [w400]
        stop <- w399 stop-if-true
        n310 = Wait (ms)(milliseconds to wait=u32 100) -> ()  [unwired: 1 out]
        n311 = call "Countdown_subVI_BM.vi"("Current Iteration"=w400, "Runtime (min)"=w401) -> ("Global Stop"=w399:bool, "Countdown Timer (min)"=w397:dbl)  [unwired: 8 in]
        n312 = global write "Elution_stop.vi" "Elution_stop"(w399) -> ()
        n313 = local write "Elution Countdown (min)"(w397) -> ()
        n314 = property class="Ctl"(reference="Elution Countdown Timer Refnum", "Value"=w397) -> (error out=w396:errorcluster)  [unwired: 1 in, 1 out]
        n315 = call <vilib>:"Clear Errors.vi"("error in (no error)"=w396) -> ()  [unwired: 5 in, 2 out]
      }
      n316 = while {
        tunnel: w385 -> [w394]
        i -> [w393]
        stop <- w391 stop-if-true
        n317 = global read "Elution_stop.vi" "Elution_stop"() -> (w392:bool)
        n318 = Wait (ms)(milliseconds to wait=u32 1000) -> ()  [unwired: 1 out]
        n319 = call "Progress_bar_subVI_BM.vi"("Global Stop"=w392, "Current Iteration"=w393, "Runtime (min)"=w394) -> ("Loop Stop"=w391:bool, "Progress Bar"=w389:u8)  [unwired: 7 in]
        n320 = local write "Elution Progress Bar"(w389) -> ()
        n321 = property class="Slide"(reference="Elution Progress Bar Refnum", "Value"=w389) -> (error out=w388:errorcluster)  [unwired: 1 in, 1 out]
        n322 = call <vilib>:"Clear Errors.vi"("error in (no error)"=w388) -> ()  [unwired: 5 in, 2 out]
      }
    }
    frame #12 {
      # "Update temperatures to write to file"
      # "Trigger plot in main VI"
      n323 = global read "Temp_global_BM.vi" "Intial Temp (oC)"() -> (w405:dbl)
      n324 = global read "Temp_global_BM.vi" "Final Temp (oC)"() -> (w407:dbl)
      n325 = global read "Temp_global_BM.vi" "Max Temp (oC)"() -> (w406:dbl)
      n326 = global write "Plot_trap_heating_global_BM.vi" "Plot trap heating"(FALSE ("Plot trap heating")) -> ()
      n327 = local read "Metadata"() -> (w403:T1)
      n328 = Bundle By Name(cluster=w403, "Initial Trap Temp (oC)"=w405, "Max Trap Temp (oC)"=w406, "Final Trap Temp (oC)"=w407) -> (w404:T1)
      n329 = local write "Metadata"(w404) -> ()
    }
    frame #13 {
      # "Write data to file"
      n330 = local read "Sample Params"() -> (w411:T5)
      n331 = local read "Current Analyte"() -> (w410:string)
      n332 = local read "Mode Selection"() -> (w414:T2)
      n333 = Unbundle By Name(w411) -> ("sample volume"=w413:dbl)
      n334 = local read "Analysis Type"() -> (w415:T6)
      n335 = local read "Metadata"() -> (w412:T1)
      n336 = call "Write_metadata_subVI_BM.vi"("Analyte"=w410, "Analysis Type"=w415, "Mode Selection"=w414, "sample volume"=w413, "Metadata"=w412) -> ()  [unwired: 7 in]
    }
    frame #14 {
      # "Update elution times from writing to file"
      # "Leave valve in Position B here - if more analysis, switch back to load in the next step"
      # "Turn off fan"
      # "Turn off drying flow again"
      n337 = local read "Constants"() -> (w421:T4)
      n338 = global read "Timestamps_global.vi" "Elution Timestamp"() -> (w419:string)
      n339 = case shown="True" w424 {
        tunnel: [u32 4 ("BitNum") u32 2 ("BitNum")] -> w423
        frame False {
        }
        frame True {
        }
      }
      n340 = Unbundle By Name(w421) -> ("BoardNum"=w420:u32)
      n341 = global write "Elution_stop.vi" "Elution_stop"(FALSE ("Elution_stop")) -> ()
      n342 = case shown="True" w424 {
        tunnel: w420 -> [_ w429]
        frame False {
        }
        frame True {
          n343 = call "BM_mcDAQ_DIO_SubVI.vi"("BoardNum"=w429, "BitValue"=FALSE, "BitNum"=u32 4) -> ("Control out"=w428:bool)  [unwired: 8 in]
          n344 = local write "Drying Flow"(w428) -> ()
        }
      }
      n345 = local read "Metadata"() -> (w417:T1)
      n346 = Bundle By Name(cluster=w417, "Elution Timestamp"=w419) -> (w418:T1)
      n347 = call "BM_mcDAQ_DIO_SubVI.vi"("BoardNum"=w420, "BitValue"=FALSE, "BitNum"=w423) -> ()  [unwired: 8 in, 1 out]
      n348 = local write "Metadata"(w418) -> ()
    }
    frame #15 {
      n349 = local read "Sample Params"() -> (w433:T5)
      n350 = Unbundle By Name(w433) -> ("Extra Burn-off"=w432:bool)
      n351 = case shown="True" w432 {
        frame False {
        }
        frame True {
          n352 = flat-sequence {
            tunnel: [w436] -> w435
            tunnel: [w445] -> w434
            tunnel: w435 -> [w445]
            tunnel: w434 -> [w452]
            frame #0 {
              # "Turn front panel indicator on"
              # "Apply heat test - does trap heat correctly?"
              n353 = local read "Constants"() -> (w440:T4)
              n354 = local read "Sample Params"() -> (w442:T5)
              n355 = Unbundle By Name(w442) -> ("Trap Heating Time (ms)"=w443:dbl)
              n356 = local read "Error in"() -> (w437:errorcluster)
              n357 = Unbundle By Name(w440) -> ("BoardNum"=w441:u32, "BitNum (Thermocouple)"=w444:u32)
              n358 = local write "Heating"(TRUE ("Heating")) -> ()
              n359 = call "BM_heat_test_subVI.vi"("error in (no error)"=w437, "Heat Pulse Delay (ms)"=u32 1000, "Trap Heating Time (ms)"=w443, "BitNum"=w444, "BoardNum"=w441) -> ("error out"=w436:errorcluster)  [unwired: 6 out]
            }
            frame #1 {
              # "Set valve to inject (pos B)"
              n360 = local read "Constants"() -> (w450:T4)
              n361 = Unbundle By Name(w450) -> ("PosA BitNum"=w449:u32, "PosB BitNum"=w448:u32, "BoardNum"=w447:u32)
              n362 = call "Switch_Valco_6port_subVI_BM.vi"("Load (T) or Inject (F)"=FALSE, "PosA BitNum"=w449, "PosB BitNum"=w448, "BoardNum"=w447) -> ()  [unwired: 6 in, 1 out]
            }
            frame #2 {
              # "Loop to heat trap - pulsing timer can be changed to modulate heating"
              n363 = local read "Constants"() -> (w451:T4)
              n364 = Unbundle By Name(w451) -> ("Heating Iterations"=w453:i32)
              n365 = for {
                N: w453 -> [_]
                tunnel: w452 -> [w457]
                n366 = flat-sequence {
                  tunnel: [w462] -> w455
                  tunnel: [w460] -> w454
                  tunnel: w457 -> [w462]
                  tunnel: [w466] -> w456
                  tunnel: w455 -> [w466]
                  tunnel: w454 -> [w465]
                  tunnel: w456 -> [w469]
                  frame #0 {
                    # "Apply current"
                    n367 = local read "Constants"() -> (w461:T4)
                    n368 = local read "Sample Params"() -> (w458:T5)
                    n369 = Unbundle By Name(w458) -> ("Trap Heating Time (ms)"=w459:dbl)
                    n370 = Unbundle By Name(w461) -> ("BoardNum"=w460:u32)
                    n371 = call "BM_mcDAQ_DIO_SubVI.vi"("BoardNum"=w460, "BitValue"=TRUE, "BitNum"=7) -> ()  [unwired: 8 in, 1 out]
                    n372 = Wait (ms)(milliseconds to wait=w459) -> ()  [unwired: 1 out]
                  }
                  frame #1 {
                    # "Stop current"
                    n373 = call "BM_mcDAQ_DIO_SubVI.vi"("BoardNum"=w465, "BitValue"=FALSE, "BitNum"=7) -> ()  [unwired: 8 in, 1 out]
                  }
                  frame #2 {
                    # "\"Pulse\" wait timer"
                    n374 = local read "Constants"() -> (w471:T4)
                    n375 = Unbundle By Name(w471) -> ("Heat Pulse Delay (ms)"=w470:dbl)
                    n376 = local write "Error out"(w469) -> ()
                    n377 = Wait (ms)(milliseconds to wait=w470) -> ()  [unwired: 1 out]
                  }
                }
              }
            }
            frame #3 {
              # "Cool the trap"
              n378 = flat-sequence {
                tunnel: [w475] -> w474
                tunnel: w474 -> [w493]
                tunnel: [w493] -> w473
                tunnel: w473 -> [w494]
                tunnel: [w494] -> w472
                tunnel: w472 -> [w496]
                frame #0 {
                  # "Turn on fan"
                  # "Turn front panel indicator off"
                  # "Start drying flow again"
                  n379 = local read "Constants"() -> (w480:T4)
                  n380 = Unbundle By Name(w480) -> ("BoardNum"=w481:u32)
                  n381 = Equal?(x=w481, y=u32 1) -> (x = y?=w475:bool)
                  n382 = case shown="True" w475 {
                    tunnel: w481 -> [_ w485]
                    frame False {
                    }
                    frame True {
                      n383 = call "BM_mcDAQ_DIO_SubVI.vi"("BoardNum"=w485, "BitValue"=TRUE, "BitNum"=u32 4) -> ("Control out"=w484:bool)  [unwired: 8 in]
                      n384 = local write "Drying Flow"(w484) -> ()
                    }
                  }
                  n385 = case shown="True" w475 {
                    tunnel: [u32 4 ("BitNum") u32 2 ("BitNum")] -> w478
                    frame False {
                    }
                    frame True {
                    }
                  }
                  n386 = local write "Heating"(FALSE ("Heating")) -> ()
                  n387 = call "BM_mcDAQ_DIO_SubVI.vi"("BoardNum"=w481, "BitValue"=TRUE, "BitNum"=w478) -> ()  [unwired: 8 in, 1 out]
                }
                frame #1 {
                  # "wait to turn off fan - equal to elution time, but don't need the progress bars in this case."
                  n388 = Multiply(x=1.5, y=60.0) -> (x*y=w490:dbl)
                  n389 = Multiply(x=w490, y=1000.0) -> (x*y=w488:dbl)
                  n390 = Wait (ms)(milliseconds to wait=w488) -> ()  [unwired: 1 out]
                }
                frame #2 {
                  # "Trigger plot in main VI"
                  n391 = global write "Plot_trap_heating_global_BM.vi" "Plot trap heating"(FALSE ("Plot trap heating")) -> ()
                }
                frame #3 {
                  # "Turn off fan"
                  # "Turn off drying flow again"
                  n392 = local read "Constants"() -> (w499:T4)
                  n393 = case shown="True" w496 {
                    tunnel: [u32 4 ("BitNum") u32 2 ("BitNum")] -> w500
                    frame False {
                    }
                    frame True {
                    }
                  }
                  n394 = Unbundle By Name(w499) -> ("BoardNum"=w498:u32)
                  n395 = case shown="True" w496 {
                    tunnel: w498 -> [_ w504]
                    frame False {
                    }
                    frame True {
                      n396 = call "BM_mcDAQ_DIO_SubVI.vi"("BoardNum"=w504, "BitValue"=FALSE, "BitNum"=u32 4) -> ("Control out"=w503:bool)  [unwired: 8 in]
                      n397 = local write "Drying Flow"(w503) -> ()
                    }
                  }
                  n398 = call "BM_mcDAQ_DIO_SubVI.vi"("BoardNum"=w498, "BitValue"=FALSE, "BitNum"=w500) -> ()  [unwired: 8 in, 1 out]
                }
              }
            }
          }
        }
      }
    }
  }
  n399 = flat-sequence {
    tunnel: w2 -> [w508]
    tunnel: w1 -> [w507]
    frame #0 {
      n400 = Wait on Notification(notifier=w508, error in (no error)=w507) -> (notifier out=w509:refnum<notifier>, error out=w510:errorcluster)  [unwired: 1 in, 3 out]
      n401 = Release Notifier(notifier=w509, error in (no error)=w510) -> ()  [unwired: 1 in, 3 out]
    }
    frame #1 {
      # "Rinse the sparger and syringe"
      n402 = local read "Constants"() -> (w520:T4)
      n403 = local read "Sample Params"() -> (w519:T5)
      n404 = local read "Pump Parameters"() -> (w517:T3)
      n405 = Unbundle By Name(w520) -> ("step to ml"=w515:dbl, "Extra Milli-Q (ml)"=w514:dbl, "N rinses"=w513:i32, "N syringe rinses"=w512:i32)
      n406 = Unbundle By Name(w519) -> ("sample volume"=w516:dbl, "Total Vol. (mL)"=w511:dbl)
      n407 = Unbundle By Name(w519) -> ("COM Port (Runze)"=w518:refnum<visa-resource-name>)
      n408 = call "Sparger_syringe_rinsing_subVI_BM.vi"("N syringe rinses"=w512, "COM Port"=w518, "N sparge rinses"=w513, "Pump Parameters"=w517, "Extra Milli-Q (ml)"=w514, "step to ml"=w515, "Total Vol. (mL)"=w511, "Sample Volume"=w516) -> ()  [unwired: 4 in]
    }
  }
  n409 = flat-sequence {
    tunnel: w6 -> [w522]
    tunnel: w5 -> [w521]
    frame #0 {
      n410 = Wait on Notification(notifier=w522, error in (no error)=w521) -> (notifier out=w524:refnum<notifier>, error out=w523:errorcluster)  [unwired: 4 out]
      n411 = Release Notifier(notifier=w524, error in (no error)=w523) -> ()  [unwired: 1 in, 3 out]
    }
    frame #1 {
      # "Read thermocouple and send to main VI"
      n412 = while {
        stop <- w527 stop-if-true
        n413 = local read "Constants"() -> (w532:T4)
        n414 = Unbundle By Name(w532) -> ("BoardNum"=w533:u32, "BitNum (Thermocouple)"=w534:u32)
        n415 = call "MC_DAQ_thermocouple_BM_subVI.vi"("BitNum"=w534, "BoardNum"=w533) -> ("Temp (oC)"=w531:dbl)  [unwired: 8 in, 1 out]
        n416 = local write "Temp (oC)"(w531) -> ()
        n417 = global read "Plot_trap_heating_global_BM.vi" "Plot trap heating"() -> (w528:bool)
        n418 = local read "Temp Refnum"() -> (w530:refnum<vi>)
        n419 = property class="Ctl"(reference=w530, "Value"=w531) -> (error out=w529:errorcluster)  [unwired: 1 in, 1 out]
        n420 = Equal?(x=w528, y=FALSE) -> (x = y?=w527:bool)
        n421 = Wait (ms)(milliseconds to wait=u32 100) -> ()  [unwired: 1 out]
        n422 = call <vilib>:"Clear Errors.vi"("error in (no error)"=w529) -> ()  [unwired: 5 in, 2 out]
      }
    }
  }
